vi "ips120 get target field.vi"(0 "VISA resource name":refnum<visa-resource-name>, 1 "error in (no error)":errorcluster) -> (2 "VISA resource name":refnum<visa-resource-name>, 3 "target field (T)":dbl, 4 "error out":errorcluster)   [LabVIEW 2013]
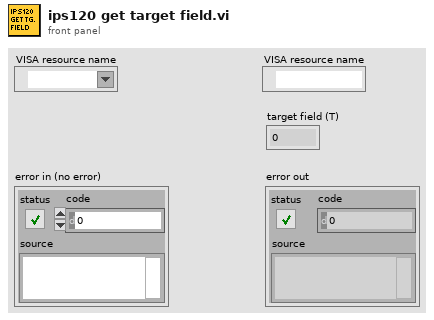
[diagram p1: front panel]
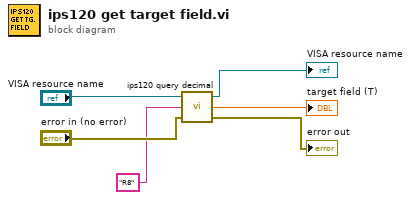
[diagram p0: block diagram]
diagram:
  n1 = call "ips120 query decimal.vi"("error in (no error)"="error in (no error)", "query"="R8", "VISA resource name"="VISA resource name") -> ("error out"=→"error out":errorcluster, "response"=→"target field (T)":dbl, "VISA resource name 2"=→"VISA resource name":refnum<visa-resource-name>)
